vi "CoolingOvershootTest.vi"(6 "Read Field":bool, 7 "Read Fan":bool, 9 "Cluster":T2, 11 "Ports":T1={"Watlows"="COM1", "Field"="COM9", "Fan"="COM4", "Flow"="COM3"}) -> (0 "Fan on":bool, 3 "Field on":bool, 4 "Run complete":bool, 5 "Current SP":dbl=50.0)   [LabVIEW 2009]
panel:
  # "Input"
  # "Output"
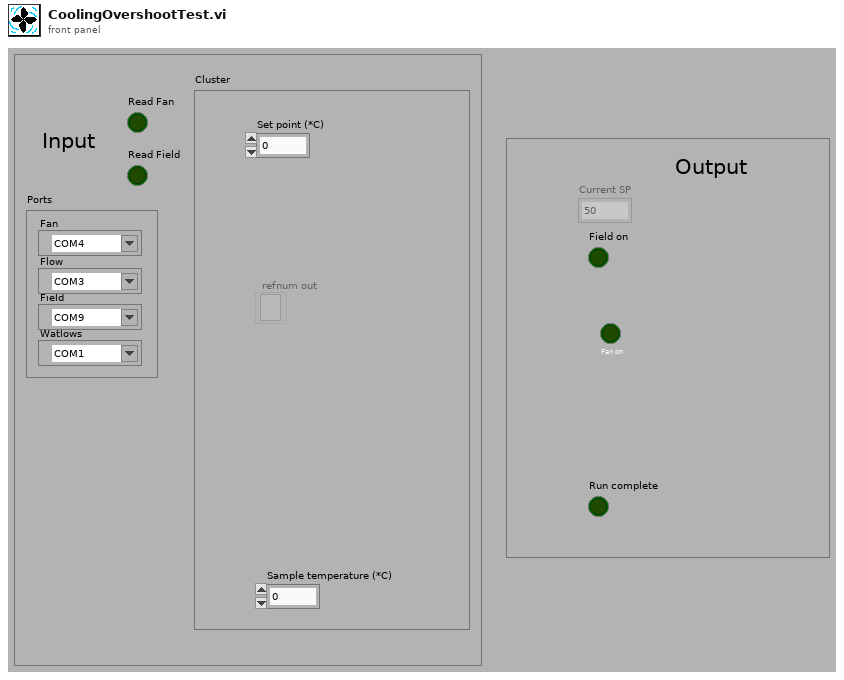
[diagram p1: front panel]
types:
  T1 = cluster{"Watlows":refnum<visa-resource-name>, "Field":refnum<visa-resource-name>, "Fan":refnum<visa-resource-name>, "Flow":refnum<visa-resource-name>}
  T2 = cluster{"Set point (*C)":u32, "Sample temperature (*C)":u32, "refnum out":refnum<file>}
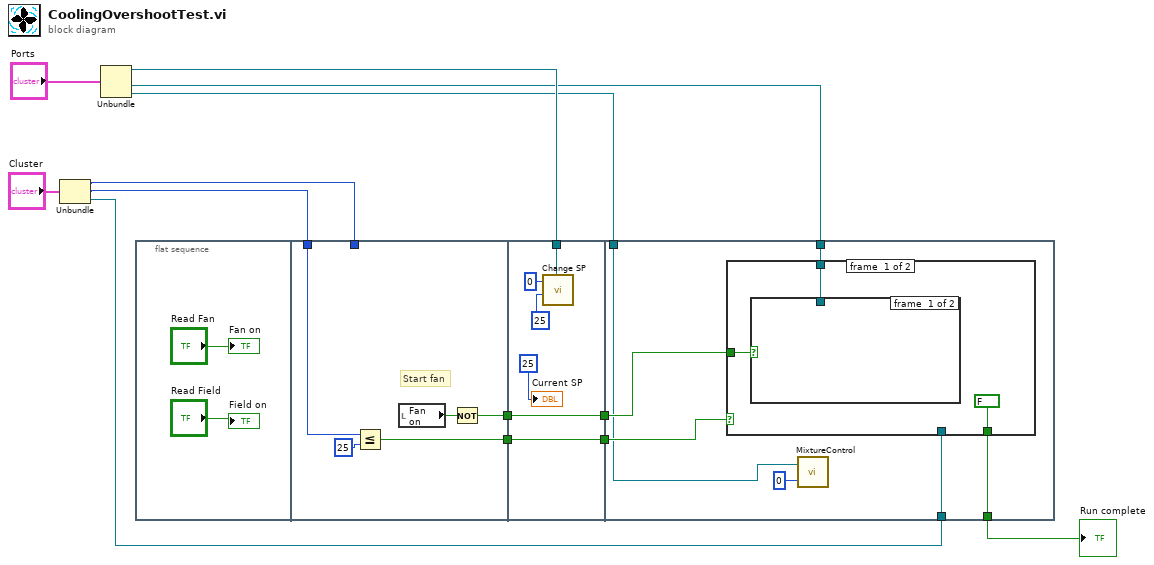
[diagram p0: block diagram]
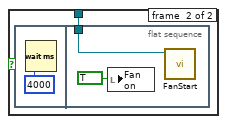
[diagram p2: hidden frame]
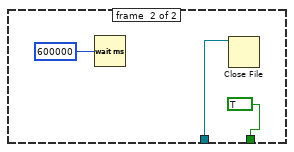
[diagram p3: hidden frame]
diagram:
  n1 = Unbundle("Cluster") -> ("Set point (*C)"=w10:u32, "Sample temperature (*C)"=w9:u32, "refnum out"=w7:refnum<file>)
  n2 = Unbundle("Ports") -> ("Watlows"=w3:refnum<visa-resource-name>, "Fan"=w2:refnum<visa-resource-name>, "Flow"=w1:refnum<visa-resource-name>)  [unwired: 1 out]
  n3 = flat-sequence {
    tunnel: w10 -> [_]
    tunnel: w9 -> [w19]
    tunnel: [w17] -> w12
    tunnel: [w16] -> w11
    tunnel: w3 -> [w24]
    tunnel: [w23] -> w6
    tunnel: w12 -> [w23]
    tunnel: w11 -> [w22]
    tunnel: [w22] -> w5
    tunnel: w7 -> [w33]
    tunnel: [w32] -> w13
    tunnel: w2 -> [w31]
    tunnel: w1 -> [w27]
    tunnel: w6 -> [w30]
    tunnel: w5 -> [w29]
    frame #0 {
      "Fan on" <- "Read Fan"
      "Field on" <- "Read Field"
    }
    frame #1 {
      # "Start fan"
      n4 = Less Or Equal?(x=w19, y=25) -> (x <= y?=w17:bool)
      n5 = local read "Fan on"() -> (w18:bool)
      n6 = Not(x=w18) -> (.not. x?=w16:bool)
    }
    frame #2 {
      n7 = call "Change SP.vi"("Set Point"=25, "Adress"=0, "VISA resource name"=w24) -> ()  [unwired: 1 in, 1 out]
      "Current SP" <- 25
    }
    frame #3 {
      n8 = case shown="False" w30 {
        tunnel: w33 -> [_ w43]
        tunnel: w29 -> [w36 _]
        tunnel: [FALSE TRUE] -> w32
        tunnel: w31 -> [w34 _]
        frame #0 {
          n9 = case shown="False" w36 {
            tunnel: w34 -> [_ w37]
            frame #0 {
            }
            frame #1 {
              n10 = flat-sequence {
                tunnel: w37 -> [w39]
                frame #0 {
                  n11 = Wait (ms)(milliseconds to wait=4000) -> ()  [unwired: 1 out]
                }
                frame #1 {
                  n12 = local write "Fan on"(TRUE) -> ()
                  n13 = call "FanStart.vi"("VISA resource name"=w39) -> ()  [unwired: 11 in]
                }
              }
            }
          }
        }
        frame #1 {
          n14 = Wait (ms)(milliseconds to wait=600000) -> ()  [unwired: 1 out]
          n15 = Close File(refnum=w43) -> ()  [unwired: 1 in, 2 out]
        }
      }
      n16 = call "MixtureControl.vi"("%CO2"=0, "VISA resource name"=w27) -> ()  [unwired: 1 in]
    }
  }
  "Run complete" <- w13
